vi "RTS Save Cluster.vi"(8 "error in (no error)":errorcluster, 9 "RTS Config Setup Save Loop":T2, 10 "CSV Data Save Loop":T11, 11 "Custom Saved Title Save Loop":T1) -> (0 "error out":errorcluster, 3 "CSV Data Save Output":T11)   [LabVIEW 2016]
uses:
  Type Definitions/RTS TDMS Filename Locations.ctl
  Type Definitions/RTS Save References.ctl
  Type Definitions/RTS Configuration Setup.ctl
  Type Definitions/RTS Wago Config.ctl
  Type Definitions/RTS APLUS Config.ctl
  Type Definitions/RTS Yokogawa MX Config.ctl
  Type Definitions/RTS Replay Server Control.ctl
  Type Definitions/RTS Server Configuration.ctl
  Type Definitions/RTS Station Settions TCP Comms.ctl
  Type Definitions/RTS Chamber Save Status.ctl
  Type Definitions/RTS Test Pattern.ctl
  Type Definitions/RTS Save Titles.ctl
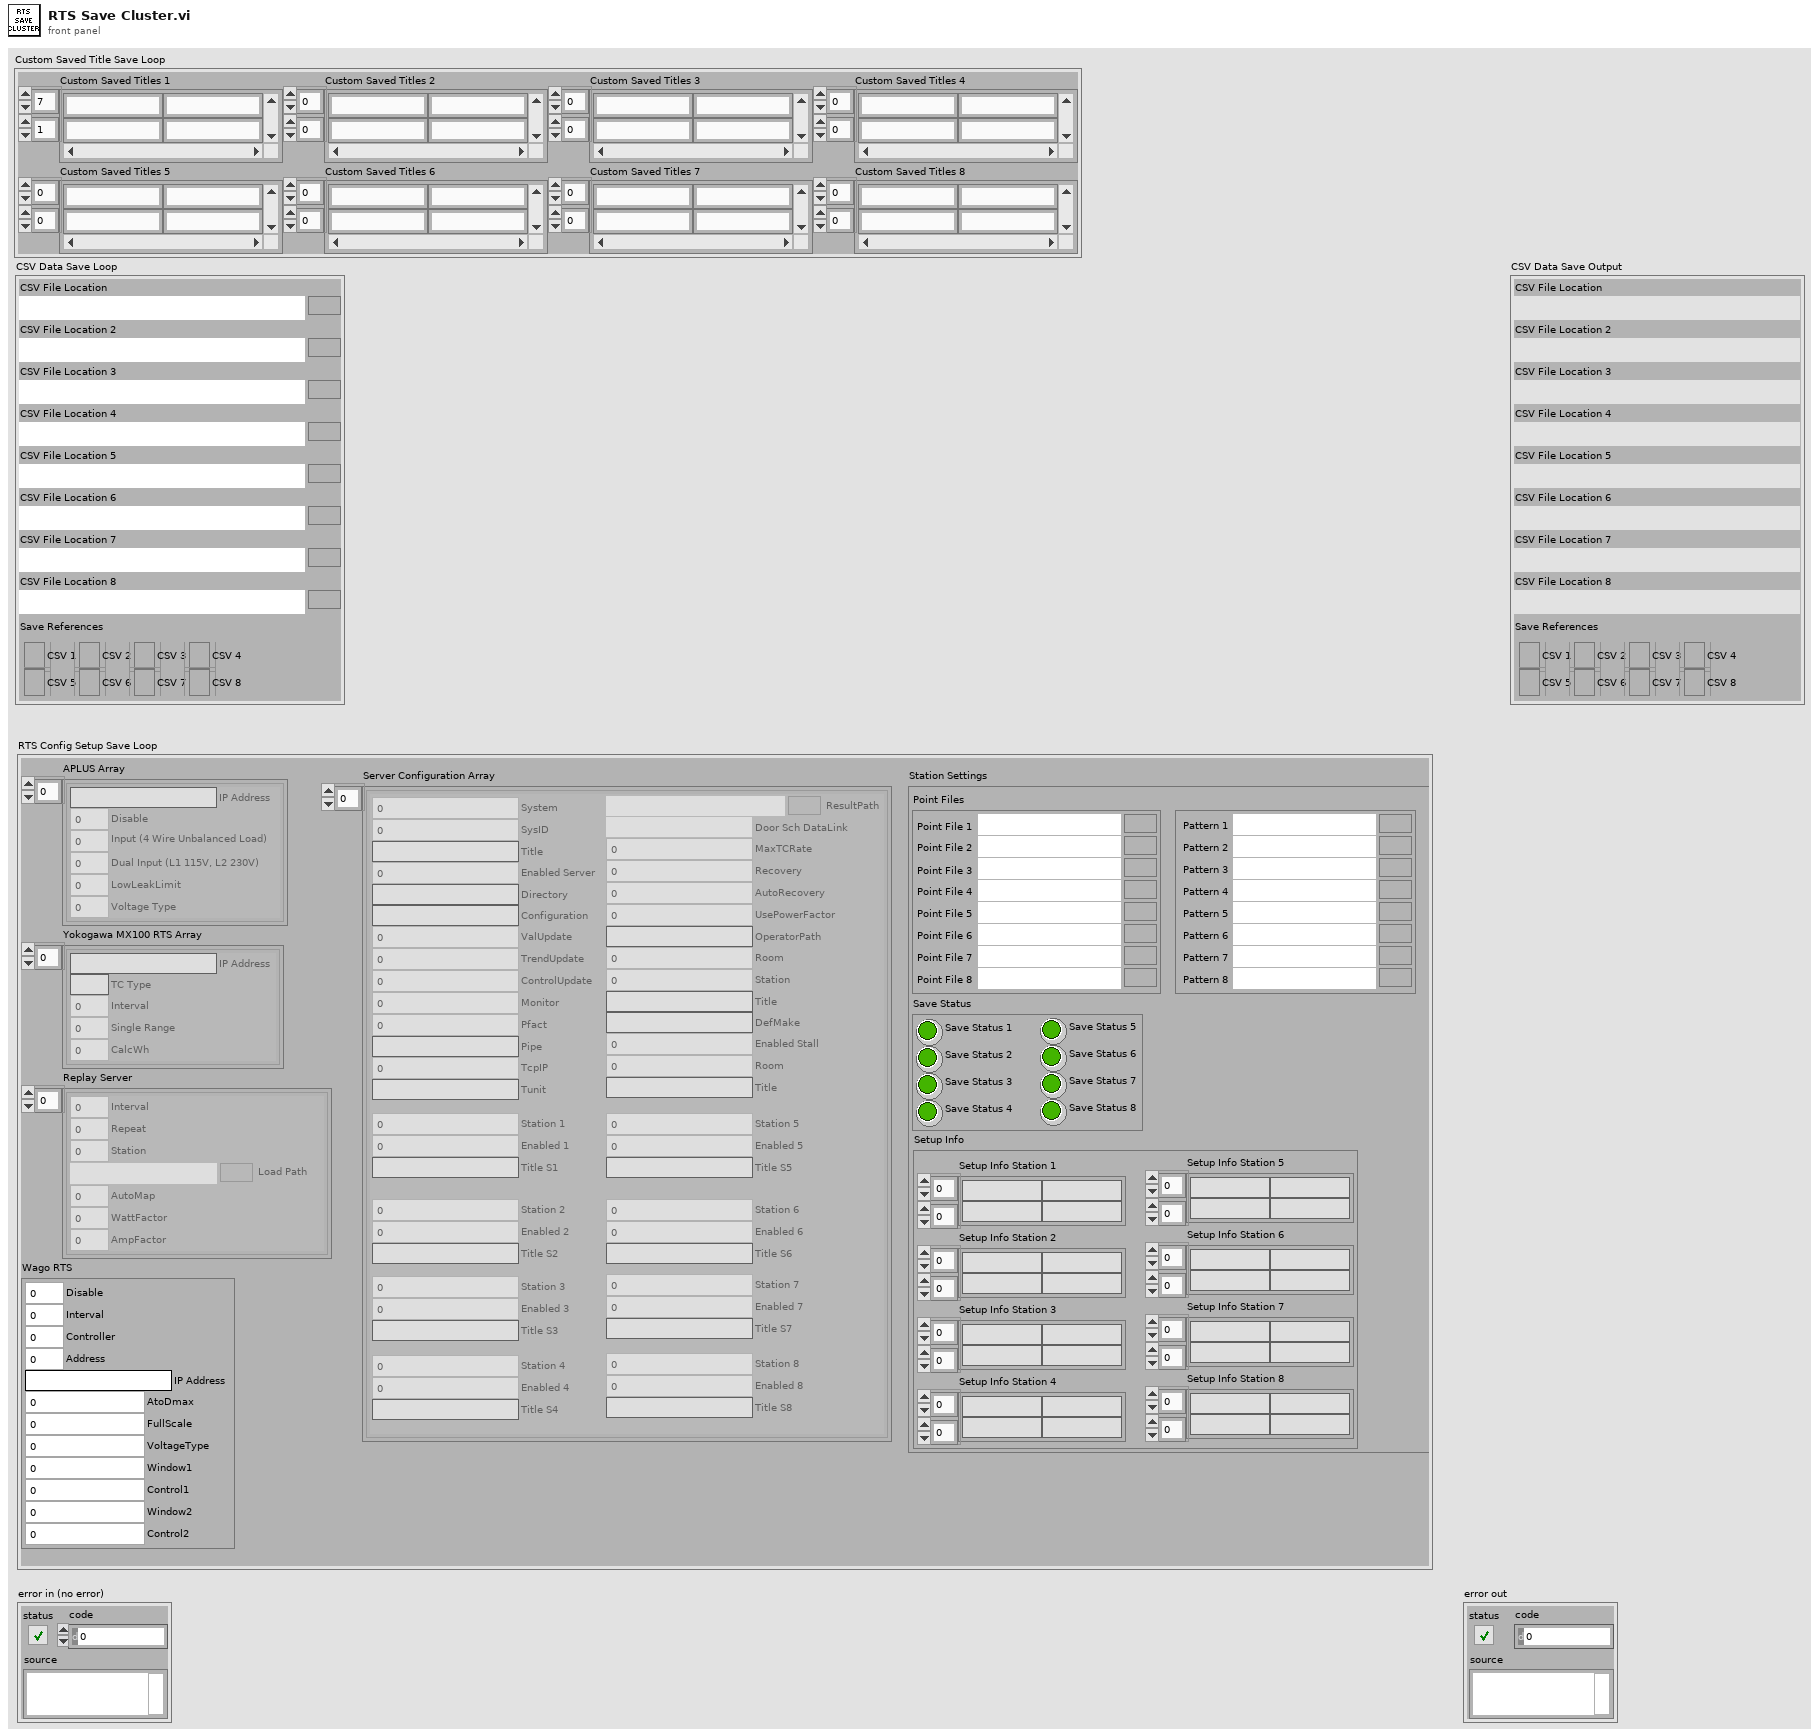
[diagram p1: front panel]
types:
  T1 = typedef "RTS Save Titles.ctl" = cluster{"Custom Saved Titles 1":string[][], "Custom Saved Titles 2":string[][], "Custom Saved Titles 3":string[][], "Custom Saved Titles 4":string[][], "Custom Saved Titles 5":string[][], "Custom Saved Titles 6":string[][], "Custom Saved Titles 7":string[][], "Custom Saved Titles 8":string[][]}
  T2 = typedef "RTS Configuration Setup.ctl" = cluster{"Wago RTS":T3, "APLUS Array":T4[], "Yokogawa MX100 RTS Array":T5[], "Replay Server":T6[], "Server Configuration Array":T7[], "Station Settings":T8}
  T3 = typedef "RTS Wago Config.ctl" = cluster{"Disable":u16, "Interval":u16, "Controller":u16, "Address":u16, "IP Address":string, "AtoDmax":u16, "FullScale":u16, "VoltageType":u16, "Window1":u16, "Control1":u16, "Window2":u16, "Control2":u16}
  T4 = typedef "RTS APLUS Config.ctl" = cluster{"Disable":u16, "IP Address":string, "Input (4 Wire Unbalanced Load)":u16, "Dual Input (L1 115V, L2 230V)":u16, "LowLeakLimit":dbl, "Voltage Type":u16}
  T5 = typedef "RTS Yokogawa MX Config.ctl" = cluster{"IP Address":string, "TC Type":string, "Interval":u16, "Single Range":u16, "CalcWh":u16}
  T6 = typedef "RTS Replay Server Control.ctl" = cluster{"Interval":i16, "Repeat":u16, "Station":u16, "Load Path":path, "AutoMap":u16, "WattFactor":dbl, "AmpFactor":dbl}
  T7 = typedef "RTS Server Configuration.ctl" = cluster{"System":u16, "SysID":u16, "Title":string, "Enabled Server":u16, "Directory":string, "Configuration":string, "ValUpdate":u16, "TrendUpdate":u16, "ControlUpdate":u16, "Monitor":u16, "Pfact":u16, "Pipe":string, "TcpIP":u16, "Tunit":string, "ResultPath":path, "Door Sch DataLink":path, "MaxTCRate":u16, "Recovery":u16, "AutoRecovery":u16, "UsePowerFactor":u16, "OperatorPath":string, "Room":u16, "Station":u16, "Title":string, "DefMake":string, "Enabled Stall":u16, "Room":u16, "Title":string, "Station 1":u16, "Enabled 1":u16, "Station 2":u16, "Enabled 2":u16, "Station 3":u16, "Enabled 3":u16, "Station 4":u16, "Enabled 4":u16, "Station 5":u16, "Enabled 5":u16, "Station 6":u16, "Enabled 6":u16, "Station 7":u16, "Enabled 7":u16, "Station 8":u16, "Enabled 8":u16, "Title S1":string, "Title S2":string, "Title S3":string, "Title S5":string, "Title S6":string, "Title S7":string, "Title S8":string, "Title S4":string}
  T8 = typedef "RTS Station Settions TCP Comms.ctl" = cluster{"Point Files":cluster{"Point File 1":path, "Point File 2":path, "Point File 3":path, "Point File 4":path, "Point File 5":path, "Point File 6":path, "Point File 7":path, "Point File 8":path}, "Save Status":T9, "Setup Info":cluster{"Setup Info Station 1":string[][], "Setup Info Station 2":string[][], "Setup Info Station 3":string[][], "Setup Info Station 4":string[][], "Setup Info Station 5":string[][], "Setup Info Station 6":string[][], "Setup Info Station 7":string[][], "Setup Info Station 8":string[][]}, "Chamber Test Pattern":T10}
  T9 = typedef "RTS Chamber Save Status.ctl" = cluster{"Save Status 1":bool, "Save Status 2":bool, "Save Status 3":bool, "Save Status 4":bool, "Save Status 5":bool, "Save Status 6":bool, "Save Status 7":bool, "Save Status 8":bool}
  T10 = typedef "RTS Test Pattern.ctl" = cluster{" Pattern 1":path, "Pattern 2":path, "Pattern 3":path, "Pattern 4":path, "Pattern 5":path, "Pattern 6":path, "Pattern 7":path, "Pattern 8":path}
  T11 = typedef "RTS TDMS Filename Locations.ctl" = cluster{"CSV File Location":path, "CSV File Location 2":path, "CSV File Location 3":path, "CSV File Location 4":path, "CSV File Location 5":path, "CSV File Location 6":path, "CSV File Location 7":path, "CSV File Location 8":path, "Save References":T12}
  T12 = typedef "RTS Save References.ctl" = cluster{"CSV 1":refnum<file>, "CSV 2":refnum<file>, "CSV 3":refnum<file>, "CSV 4":refnum<file>, "CSV 5":refnum<file>, "CSV 6":refnum<file>, "CSV 7":refnum<file>, "CSV 8":refnum<file>}
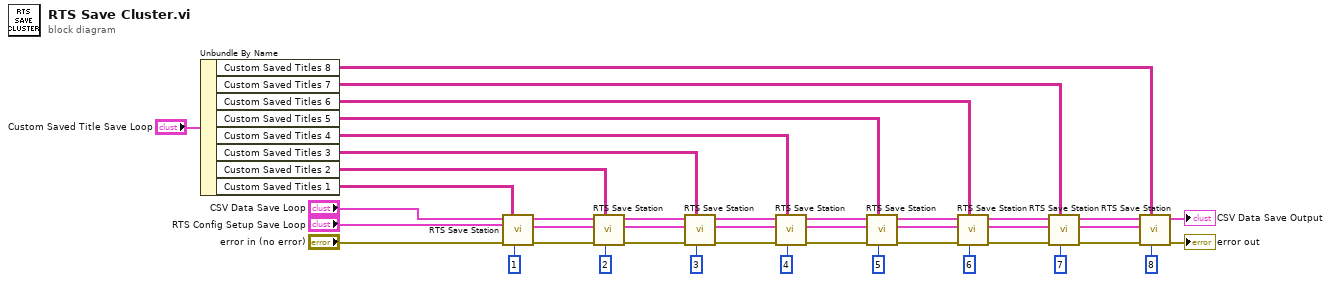
[diagram p0: block diagram]
diagram:
  n1 = Unbundle By Name("Custom Saved Title Save Loop") -> ("Custom Saved Titles 8"=w1:string[][], "Custom Saved Titles 7"=w2:string[][], "Custom Saved Titles 6"=w3:string[][], "Custom Saved Titles 5"=w4:string[][], "Custom Saved Titles 4"=w5:string[][], "Custom Saved Titles 3"=w6:string[][], "Custom Saved Titles 2"=w7:string[][], "Custom Saved Titles 1"=w8:string[][])
  n2 = call "RTS Save Station.vi"("Station Number"=u8 1, "Custom Saved Titles"=w8, "error in (no error)"="error in (no error)", "RTS Config Setup Save Loop"="RTS Config Setup Save Loop", "TDMS Data Save Loop"="CSV Data Save Loop") -> ("error out"=w28:errorcluster, "RTS Config Setup Save Loop Out"=w24:T2, "CSV Data Save Output"=w36:T11)  [unwired: 4 in]
  n3 = call "RTS Save Station.vi"("Station Number"=u8 2, "Custom Saved Titles"=w7, "error in (no error)"=w28, "RTS Config Setup Save Loop"=w24, "TDMS Data Save Loop"=w36) -> ("error out"=w29:errorcluster, "RTS Config Setup Save Loop Out"=w23:T2, "CSV Data Save Output"=w37:T11)  [unwired: 4 in]
  n4 = call "RTS Save Station.vi"("Station Number"=u8 3, "Custom Saved Titles"=w6, "error in (no error)"=w29, "RTS Config Setup Save Loop"=w23, "TDMS Data Save Loop"=w37) -> ("error out"=w30:errorcluster, "RTS Config Setup Save Loop Out"=w22:T2, "CSV Data Save Output"=w38:T11)  [unwired: 4 in]
  n5 = call "RTS Save Station.vi"("Station Number"=u8 4, "Custom Saved Titles"=w5, "error in (no error)"=w30, "RTS Config Setup Save Loop"=w22, "TDMS Data Save Loop"=w38) -> ("error out"=w31:errorcluster, "RTS Config Setup Save Loop Out"=w21:T2, "CSV Data Save Output"=w39:T11)  [unwired: 4 in]
  n6 = call "RTS Save Station.vi"("Station Number"=u8 5, "Custom Saved Titles"=w4, "error in (no error)"=w31, "RTS Config Setup Save Loop"=w21, "TDMS Data Save Loop"=w39) -> ("error out"=w32:errorcluster, "RTS Config Setup Save Loop Out"=w20:T2, "CSV Data Save Output"=w40:T11)  [unwired: 4 in]
  n7 = call "RTS Save Station.vi"("Station Number"=u8 6, "Custom Saved Titles"=w3, "error in (no error)"=w32, "RTS Config Setup Save Loop"=w20, "TDMS Data Save Loop"=w40) -> ("error out"=w33:errorcluster, "RTS Config Setup Save Loop Out"=w19:T2, "CSV Data Save Output"=w41:T11)  [unwired: 4 in]
  n8 = call "RTS Save Station.vi"("Station Number"=u8 7, "Custom Saved Titles"=w2, "error in (no error)"=w33, "RTS Config Setup Save Loop"=w19, "TDMS Data Save Loop"=w41) -> ("error out"=w34:errorcluster, "RTS Config Setup Save Loop Out"=w18:T2, "CSV Data Save Output"=w42:T11)  [unwired: 4 in]
  n9 = call "RTS Save Station.vi"("Station Number"=u8 8, "Custom Saved Titles"=w1, "error in (no error)"=w34, "RTS Config Setup Save Loop"=w18, "TDMS Data Save Loop"=w42) -> ("error out"=→"error out":errorcluster, "CSV Data Save Output"=→"CSV Data Save Output":T11)  [unwired: 4 in, 1 out]
